vi "average_meas_duration.vi"(0 "current meas cycle":i32, 1 "current step":i32, 2 "time diff (ms)":u32) -> (3 "time for this step":string, 4 "step duration":string="00:00:00", 5 "time left for exp":string="00:00:00", 6 "meas cycle \nduration (s)":dbl=2.0)   [LabVIEW 2011]
uses:
  global.vi
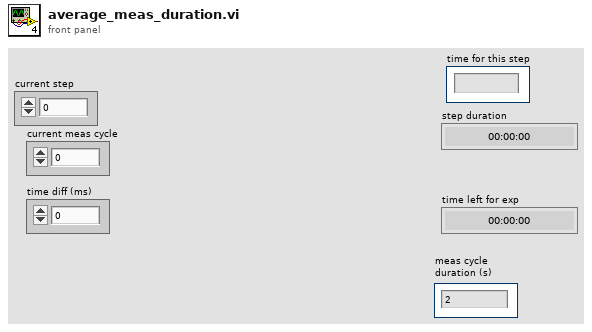
[diagram p1: front panel]
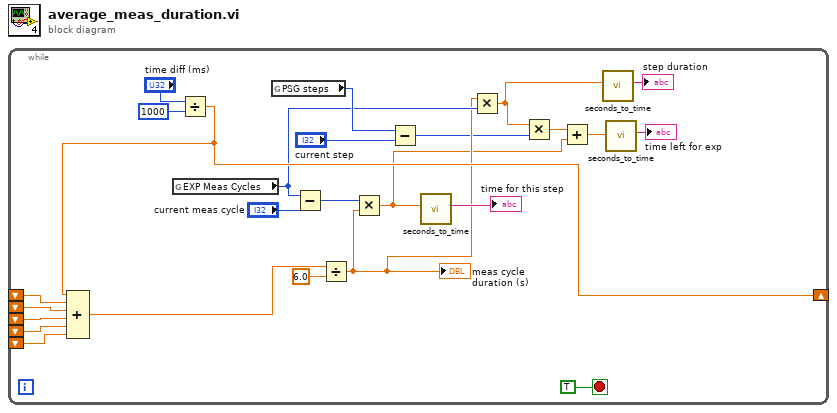
[diagram p0: block diagram]
diagram:
  n1 = while {
    shift-right: [w15] -> _
    shift-left: _ -> [w20]
    shift-left: _ -> [w19]
    shift-left: _ -> [w17]
    shift-left: _ -> [w18]
    shift-left: _ -> [w16]
    stop <- TRUE stop-if-true
    n2 = global read "global.vi" "EXP Meas Cycles"() -> (w9:i32)
    n3 = Divide(x="time diff (ms)", y=u32 1000) -> (x/y=w15:dbl)
    n4 = Compound Arithmetic op=ADD(w15, w20, w19, w18, w17, w16) -> (w14:dbl)
    n5 = global read "global.vi" "PSG steps"() -> (w11:i32)
    n6 = Subtract(x=w9, y="current meas cycle") -> (x-y=w23:i32)
    n7 = Divide(x=w14, y=6.0) -> (x/y=w8:dbl)
    "meas cycle \nduration (s)" <- w8
    n8 = Multiply(x=w23, y=w8) -> (x*y=w5:dbl)
    n9 = Subtract(x=w11, y="current step") -> (x-y=w7:i32)
    n10 = call "seconds_to_time.vi"("# Seconds (0)"=w5) -> ("Elapsed Time (00:00:00)"=→"time for this step":string)  [unwired: 10 in]
    n11 = Multiply(x=w8, y=w9) -> (x*y=w2:dbl)
    n12 = Multiply(x=w2, y=w7) -> (x*y=w6:dbl)
    n13 = Add(x=w6, y=w5) -> (x+y=w4:dbl)
    n14 = call "seconds_to_time.vi"("# Seconds (0)"=w2) -> ("Elapsed Time (00:00:00)"=→"step duration":string)  [unwired: 10 in]
    n15 = call "seconds_to_time.vi"("# Seconds (0)"=w4) -> ("Elapsed Time (00:00:00)"=→"time left for exp":string)  [unwired: 10 in]
  }
